vi "GetPixelToGantryRelPosition.vi"(3 "error in (no error)":errorcluster, 4 "PixelY":dbl, 5 "PixelX":dbl) -> (0 "error out":errorcluster, 1 "YmmRelGH":dbl, 2 "XmmRelGH":dbl)   [LabVIEW 2019]
panel:
  in  "GHtoCamOffsetYmm":dbl=117.045
  in  "GHtoCamOffsetXmm":dbl=29.795
  in  "NPixelsY":dbl=1920.0
  in  "NPixelsX":dbl=2560.0
  in  "MicronsPerPixel":dbl=0.4348
  # "Convert pixels to X and Y relative to gantry head (GH). Units of X & Y are in mm."
  # "Constants here"
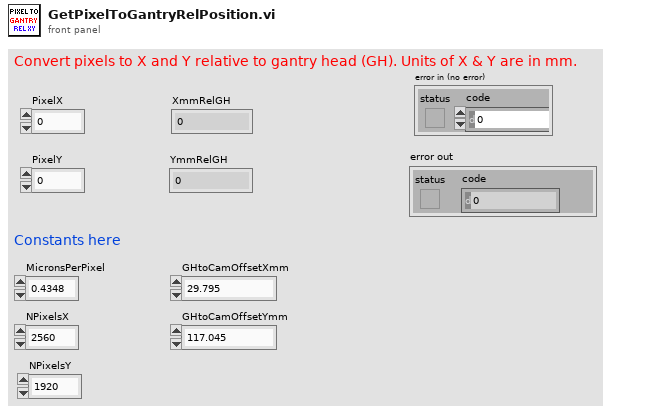
[diagram p1: front panel]
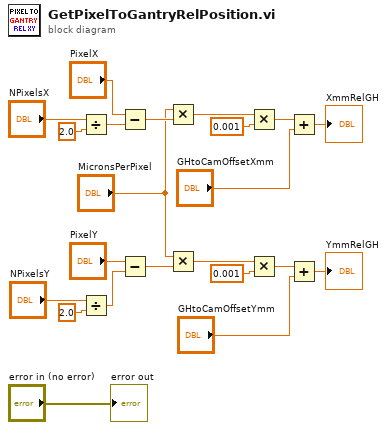
[diagram p0: block diagram]
diagram:
  n1 = Divide(x="NPixelsX", y=2.0) -> (x/y=w17:dbl)
  n2 = Divide(x="NPixelsY", y=2.0) -> (x/y=w15:dbl)
  n3 = Subtract(x="PixelX", y=w17) -> (x-y=w14:dbl)
  n4 = Subtract(x="PixelY", y=w15) -> (x-y=w13:dbl)
  n5 = Multiply(x="MicronsPerPixel", y=w14) -> (x*y=w8:dbl)
  n6 = Multiply(x="MicronsPerPixel", y=w13) -> (x*y=w6:dbl)
  n7 = Multiply(x=w8, y=0.001) -> (x*y=w2:dbl)
  n8 = Multiply(x=w6, y=0.001) -> (x*y=w3:dbl)
  n9 = Add(x=w2, y="GHtoCamOffsetXmm") -> (x+y=→"XmmRelGH":dbl)
  n10 = Add(x=w3, y="GHtoCamOffsetYmm") -> (x+y=→"YmmRelGH":dbl)
  "error out" <- "error in (no error)"
